vi "set wait.vi"(8 "error in (no error)":errorcluster, 11 "value":u16) -> (0 "error out":errorcluster)   [LabVIEW 2015, in "SCANalone4x64.lvlib"]
doc: "__declspec(dllimport) void __stdcall set_wait(unsigned short value);"
uses:
  <userlib>/SCANalone4x64/SCANalone4x64.lvlib
  <userlib>/SCANalone4x64/SCANalone4x64.dll
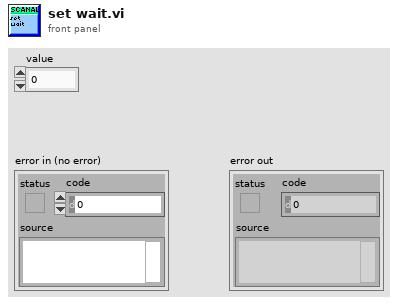
[diagram p1: front panel]
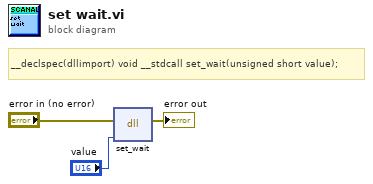
[diagram p0: block diagram]
diagram:
  # "__declspec(dllimport) void __stdcall set_wait(unsigned short value);"
  n1 = dll-call lib="C:/Program Files/National Instruments/LabVIEW 2015/user.lib/SCANalone4x64/SCANalone4x64.*" fn="set_wait"(error in="error in (no error)", "value"="value") -> (error out=→"error out":errorcluster)  [unwired: 4 in, 1 out]
